vi "_readString[]CommandArgument.vi"(7 "Error If Not Found":bool=TRUE, 8 "error in (no error)":errorcluster, 9 "Item":string, 10 "Command Spec":refnum<class "tBSONDocument.lvclass">, 11 "Main Build Spec":refnum<class "tBSONDocument.lvclass">) -> (0 "error out":errorcluster, 1 "Value":string[](array[string]), 2 "Command Spec out":refnum<class "tBSONDocument.lvclass">, 3 "Main Build Spec out":refnum<class "tBSONDocument.lvclass">)   [LabVIEW 2013, in "LVAutomationListener.lvlib" / "LVAutomationListener.lvclass"]
uses:
  LVAutomationListener.lvclass
  BSON/tBSONDocument/tBSONDocument.lvclass
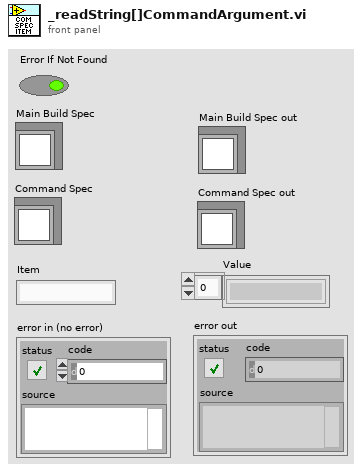
[diagram p1: front panel]
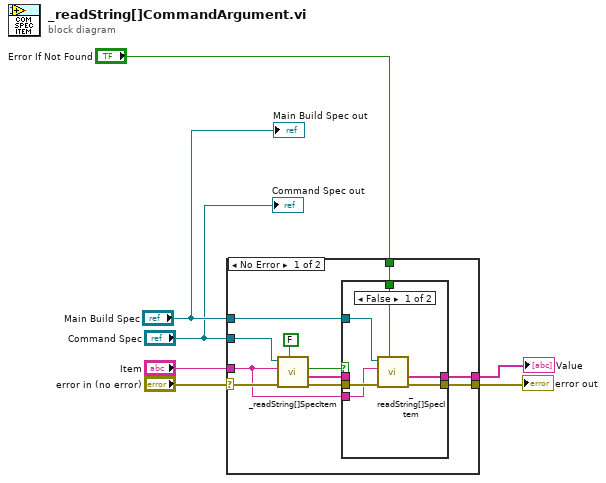
[diagram p0: block diagram]
diagram:
  n1 = case shown="No Error" "error in (no error)" {
    selector: "error in (no error)" -> [w18 w27]
    tunnel: "Item" -> [w10 _]
    tunnel: "Command Spec" -> [w16 _]
    tunnel: [w12 w27] -> w5
    tunnel: "Main Build Spec" -> [w11 _]
    tunnel: [w9 _] -> w4
    tunnel: "Error If Not Found" -> [w8 _]
    frame No Error {
      n2 = call "_readString[]SpecItem.vi"("Error If Not Found"=FALSE, "error in (no error)"=w18, "Name"=w10, "Build Spec In"=w16) -> ("error out"=w13:errorcluster, "Value"=w14:string[], "Found"=w15:bool)  [unwired: 4 in, 1 out]
      n3 = case shown="False" w15 {
        tunnel: w14 -> [_ w25]
        tunnel: w13 -> [w24 w26]
        tunnel: [w21 w26] -> w12
        tunnel: w11 -> [w22 _]
        tunnel: w10 -> [w23 _]
        tunnel: [w20 w25] -> w9
        tunnel: w8 -> [w19 _]
        frame False {
          n4 = call "_readString[]SpecItem.vi"("Error If Not Found"=w19, "error in (no error)"=w24, "Name"=w23, "Build Spec In"=w22) -> ("error out"=w21:errorcluster, "Value"=w20:string[])  [unwired: 4 in, 2 out]
        }
        frame True {
        }
      }
    }
    frame Error {
    }
  }
  "error out" <- w5
  "Value" <- w4
  "Main Build Spec out" <- "Main Build Spec"
  "Command Spec out" <- "Command Spec"
